vi "SRV_PM_Separate Extra Packet Bytes.vi"(0 "Packet":u8[](array[numeric]) format="%.0x", 9 "Total Packet Length":u16, 11 "error in (no error)":errorcluster) -> (13 "Packet Data sans Extra Bytes":u8[](array[numeric]) format="%.0x", 14 "Extra Bytes":u8[](array[numeric]) format="%.0x", 15 "error out":errorcluster)   [LabVIEW 2014]
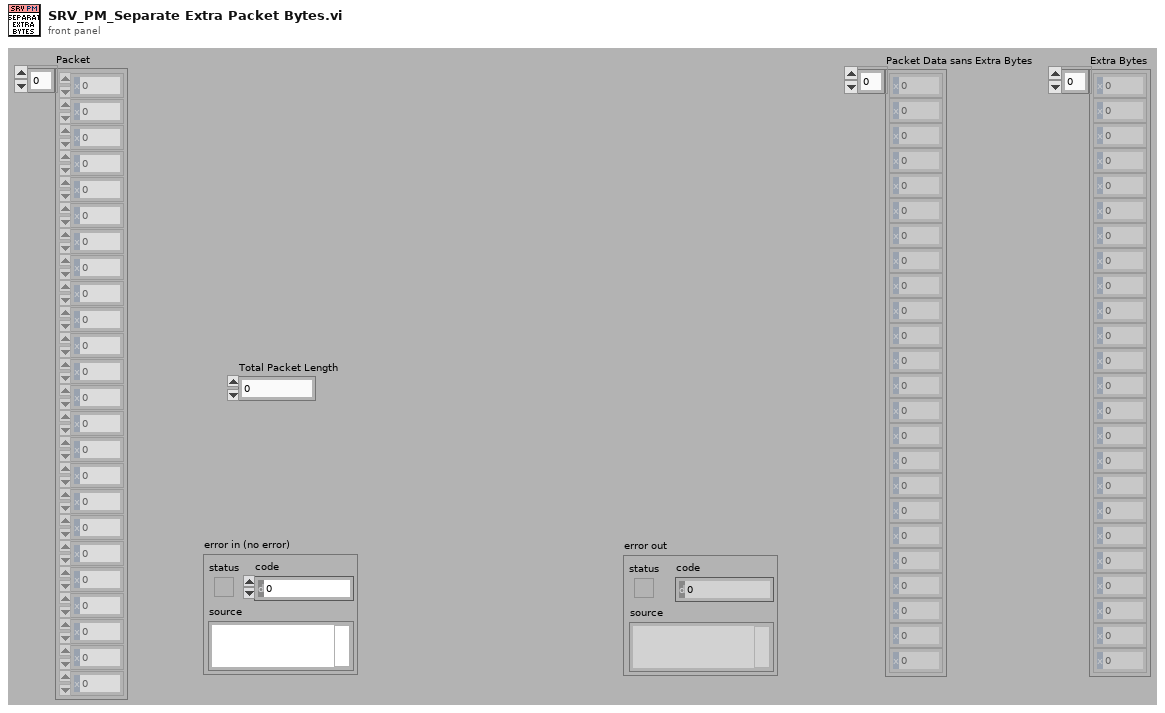
[diagram p1: front panel]
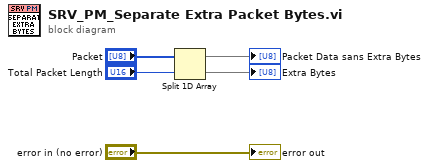
[diagram p0: block diagram]
diagram:
  n1 = Split 1D Array(array="Packet", index="Total Packet Length") -> (first subarray=→"Packet Data sans Extra Bytes":u8[], second subarray=→"Extra Bytes":u8[])
  "error out" <- "error in (no error)"
